vi "Open_Instr.vi"(8 "error in (no error)":errorcluster caption="entrée d'erreur (pas d'erreur)", 11 "Class DIO en entrée":refnum<class "Class Instrument DIO.lvclass">) -> (0 "error out":errorcluster caption="sortie d'erreur", 3 "Class DIO en Sortie":refnum<class "Class Instrument DIO.lvclass">)   [LabVIEW 2020, in "Library Instrument & Equipement.lvlib" / "Library Instruments.lvlib" / "Class Instrument DIO.lvclass"]
uses:
  Class Instrument DIO.lvclass
  Class Instrument DIO.lvclass/Class Instrument DIO.ctl
  Instrument (Default)/Class Instrument (Default).lvclass
  DIO/Class DIO (Default)/Class DIO (Default).lvclass
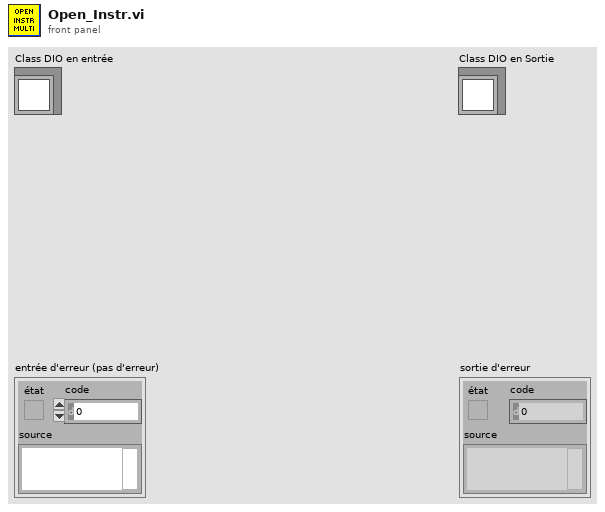
[diagram p1: front panel]
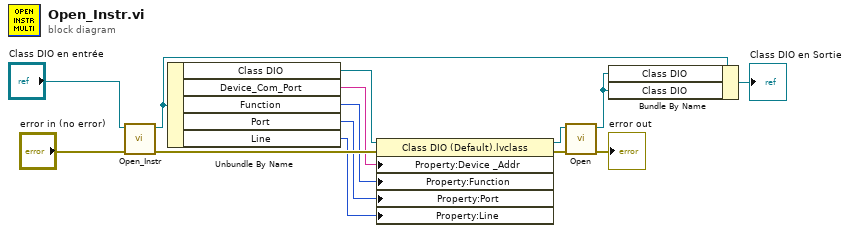
[diagram p0: block diagram]
diagram:
  n1 = call-parent "Open_Instr.vi"("error in (no error)"="error in (no error)", "Class Multimeter (Default) en entrée"="Class DIO en entrée") -> ("error out"=w12:errorcluster, "Class Multimeter (Default) en sortie"=w9:refnum<class "Class Instrument DIO.lvclass">)  [unwired: 8 in]
  n2 = Unbundle By Name(w9) -> ("Class DIO"=w11:refnum<class "Class DIO (Default).lvclass">, "Device_Com_Port"=w10:string, "Function"=w4:enum16{"Write", "Read"}, "Port"=w3:u8, "Line"=w2:u8)
  n3 = property class="Class DIO (Default).lvclass"(reference=w11, error in=w12, "Property:Device _Addr"=w10, "Property:Function"=w4, "Property:Port"=w3, "Property:Line"=w2) -> (reference out=w5:refnum<class "Class DIO (Default).lvclass">, error out=w7:errorcluster)
  n4 = call-dynamic "Open.vi"("error in (no error)"=w7, "Class DIO (Default) en entrée"=w5) -> ("error out"=→"error out":errorcluster, "Class DIO (Default) en sortie"=w1:refnum<class "Class DIO (Default).lvclass">)  [unwired: 8 in]
  n5 = Bundle By Name(cluster=w9, "Class DIO"=w1, "Class DIO"=w1) -> (→"Class DIO en Sortie":refnum<class "Class Instrument DIO.lvclass">)
